vi "Application Memory Monitor.vi"() -> ()   [LabVIEW 2016]
uses:
  <vilib>/Utility/error.llb/DialogType.ctl
  SLL Queued State Machine/Queue Driver/Create Queue.vi
  SLL Queued State Machine/Queue Driver/Enqueue an Item to Queue.vi
  SLL Queued State Machine/Queue Driver/Dequeue Queue.vi
  SLL Queued State Machine/Queue Driver/Enqueue N Items.vi
  SLL Queued State Machine/Queue Driver/Flush Queue.vi
  SLL Queued State Machine/Queue Driver/Release Queue.vi
  SLL Queued State Machine/SLL QSM.lvlib
panel:
  in  "Start":bool
  in  "Sampling Rate (s)":dbl=1.0
  in  "Application Image Name":string="LabVIEW"
  out "Waveform Chart":T1(graph)
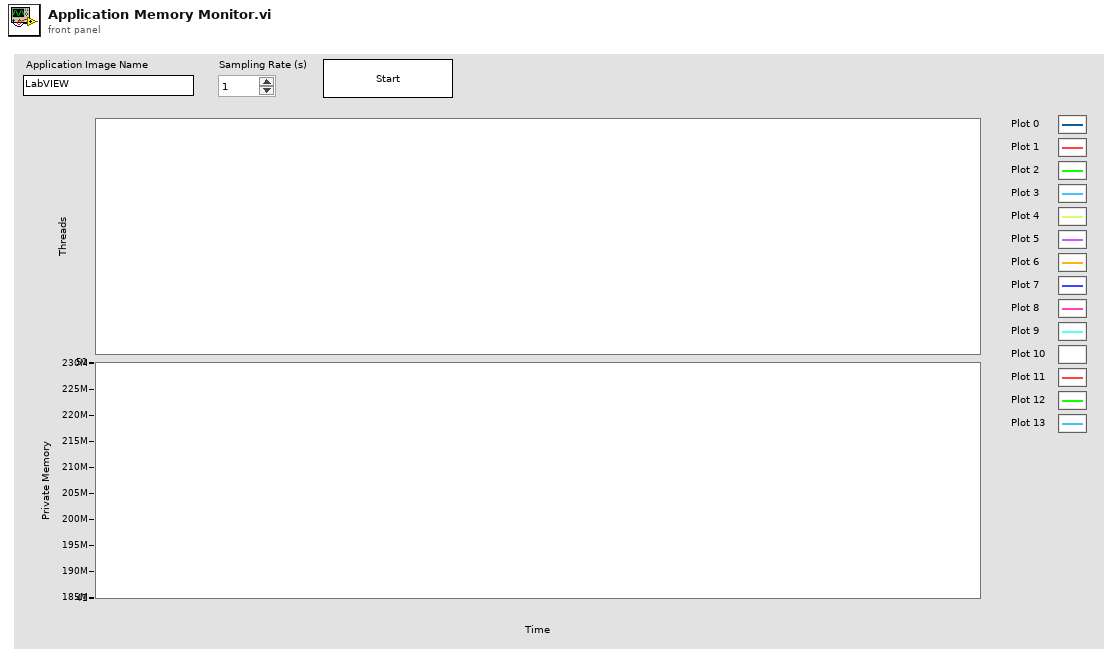
[diagram p1: front panel]
types:
  T1 = cluster{"Thread Count":i32, "PrivateMemorySize64":i64}
  T2 = cluster{"Flags":cluster{"Source Code?":bool, "Running?":bool}, "Application Name":string, "Ref":cluster{"ProcessMain":refnum<k24>, "UserProcess":refnum<k24>, "Threads":refnum<k24>}, "Sampling Rate (ms)":i32}
  T3 = cluster{"Thread Count":i32, "PrivateMemorySize64":i64}[]
  T4 = typedef "DialogType.ctl" = u16
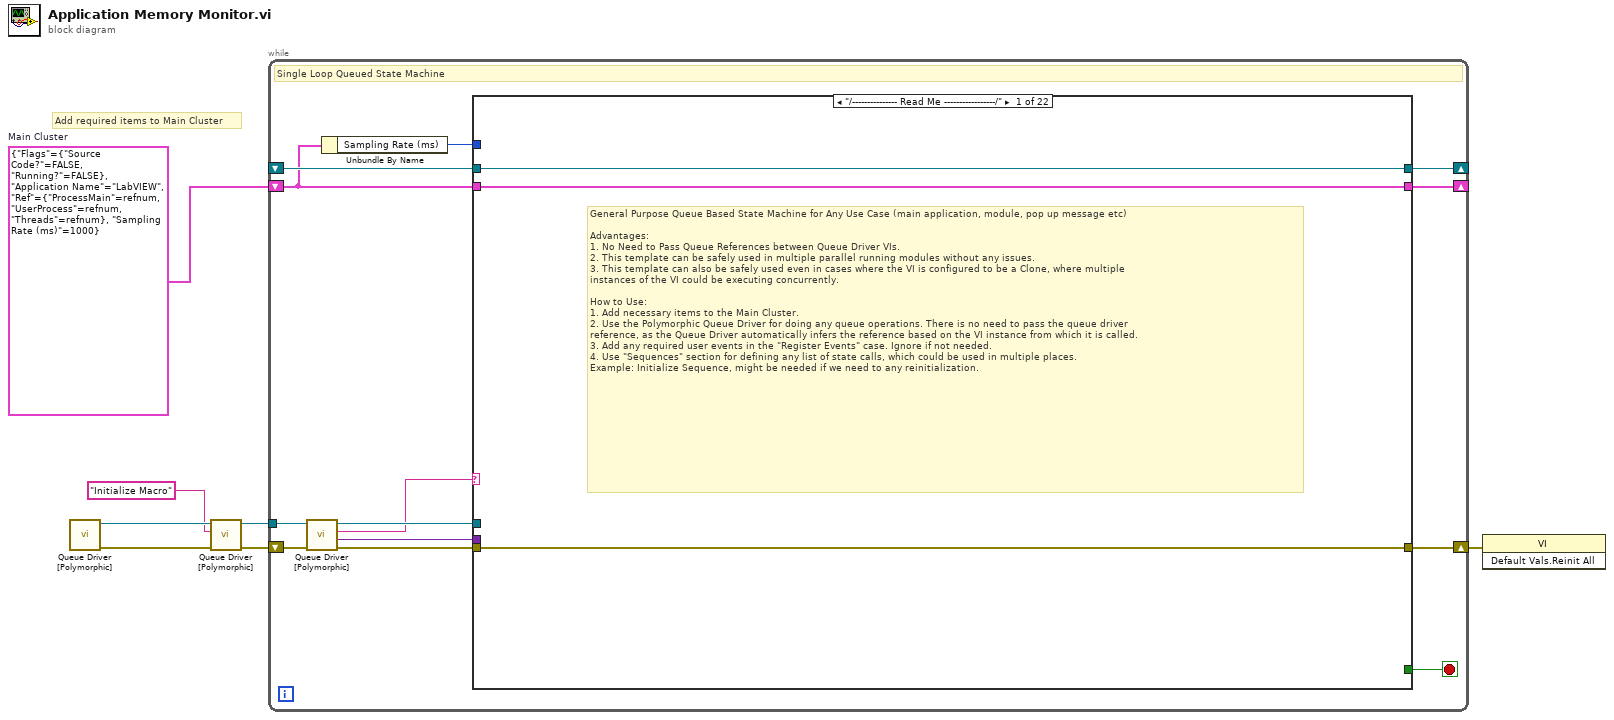
[diagram p0: block diagram]
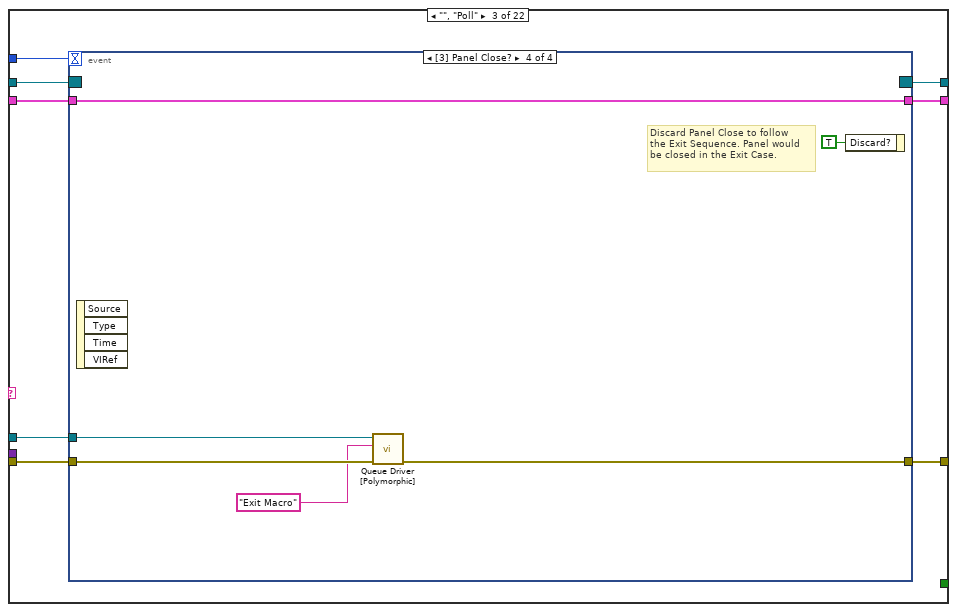
[diagram p3: hidden frame]
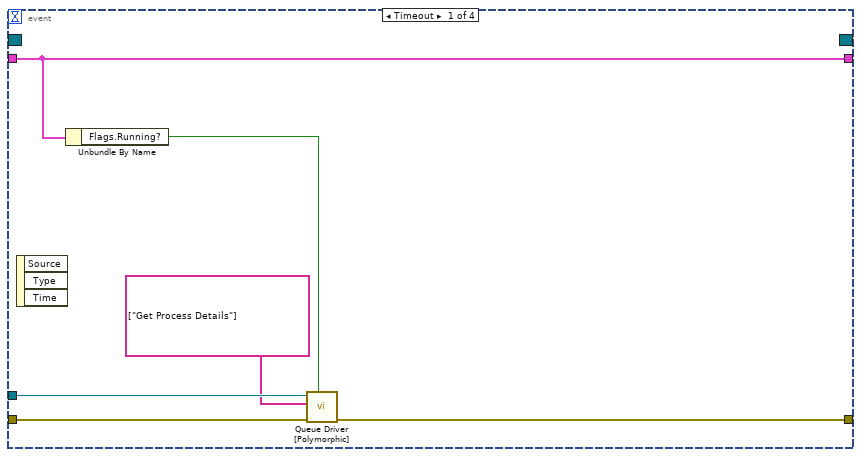
[diagram p4: hidden frame]
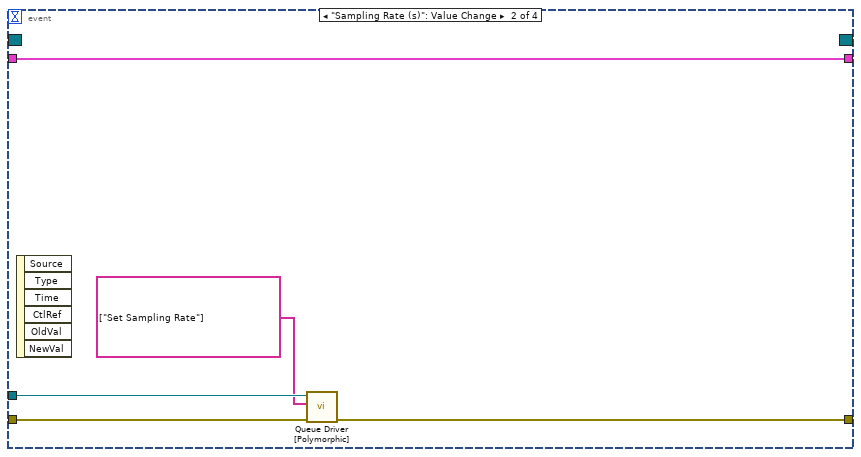
[diagram p5: hidden frame]
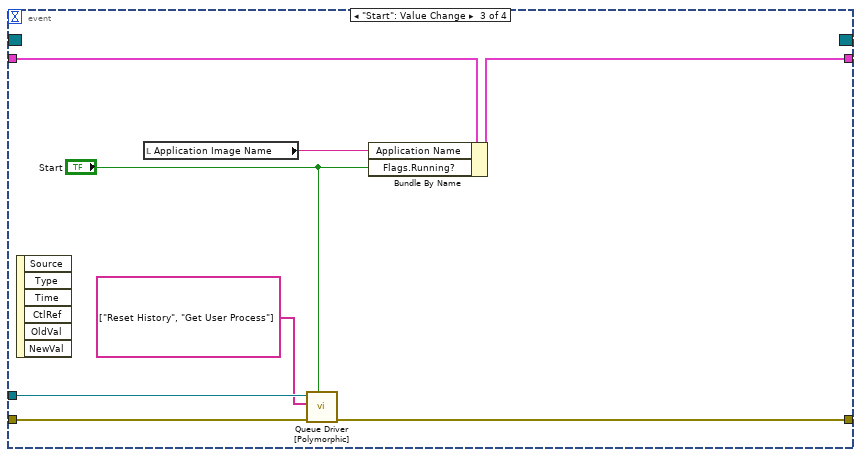
[diagram p6: hidden frame]
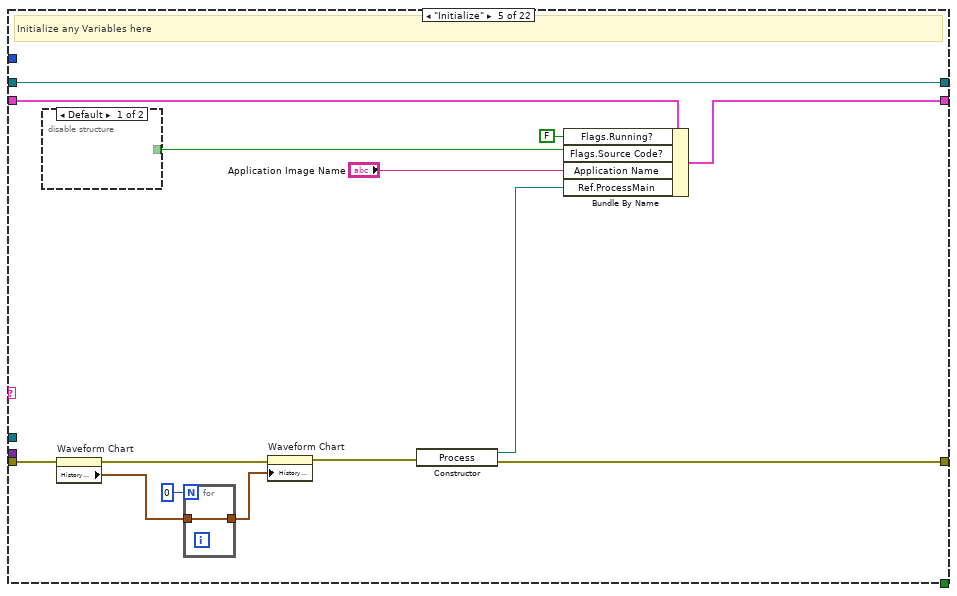
[diagram p8: hidden frame]
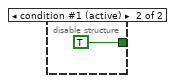
[diagram p9: hidden frame]
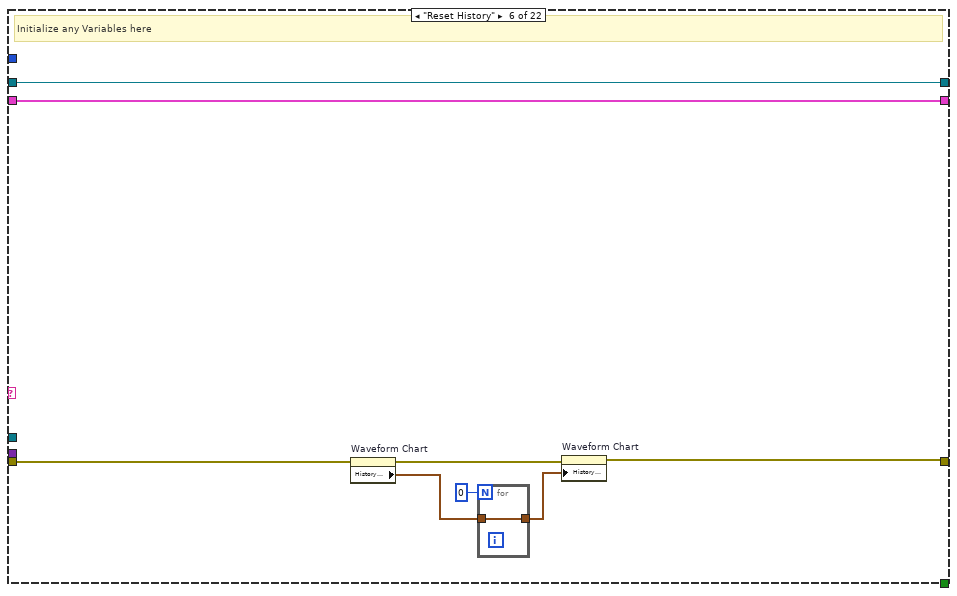
[diagram p10: hidden frame]
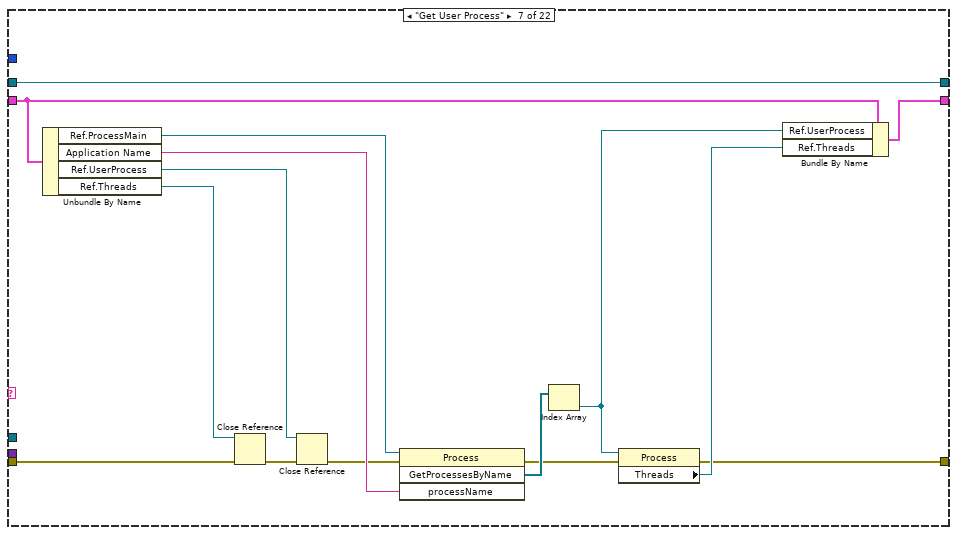
[diagram p11: hidden frame]
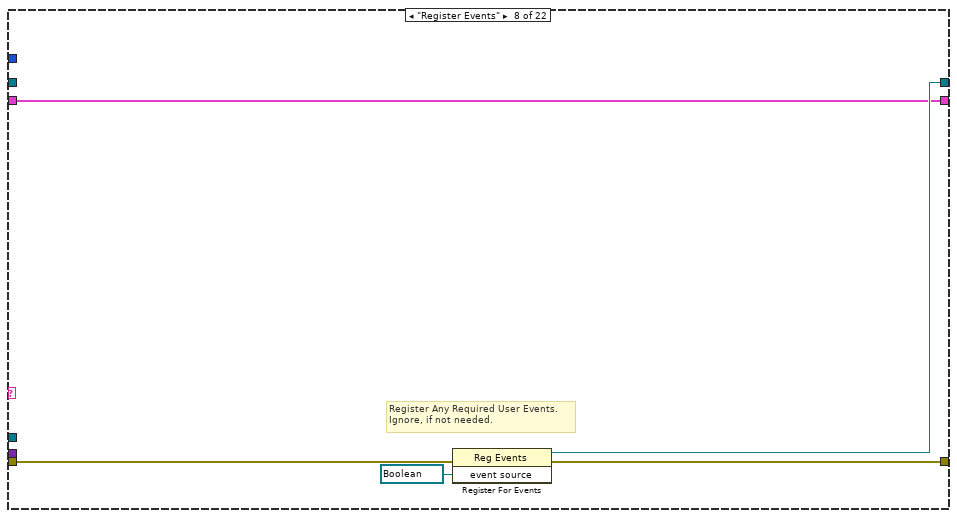
[diagram p12: hidden frame]
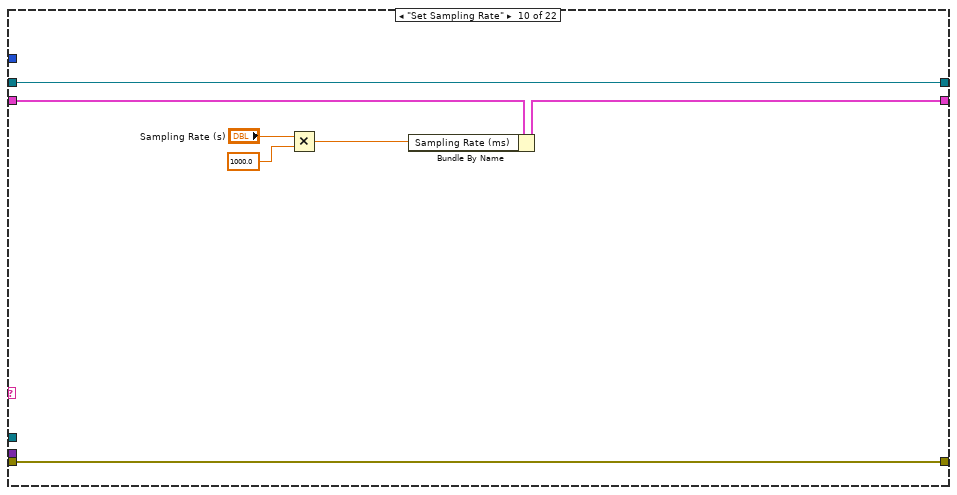
[diagram p14: hidden frame]
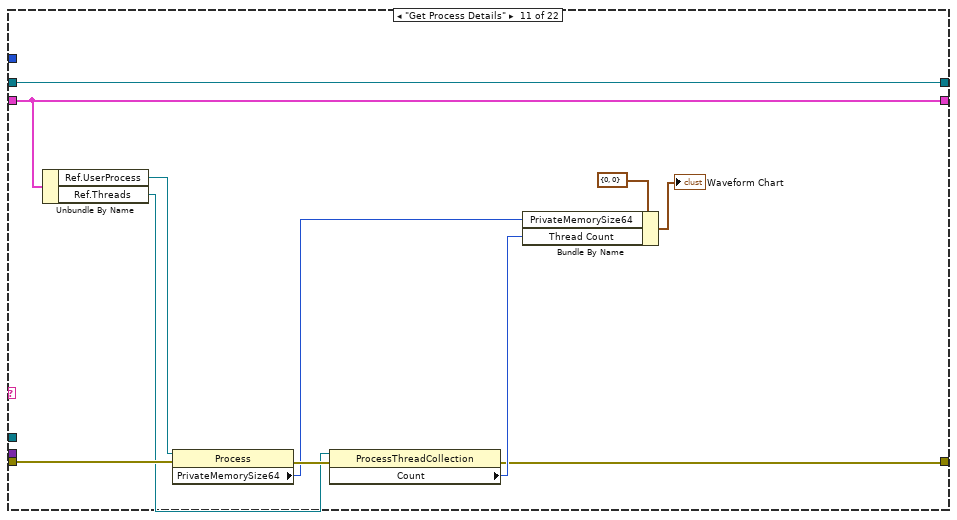
[diagram p15: hidden frame]
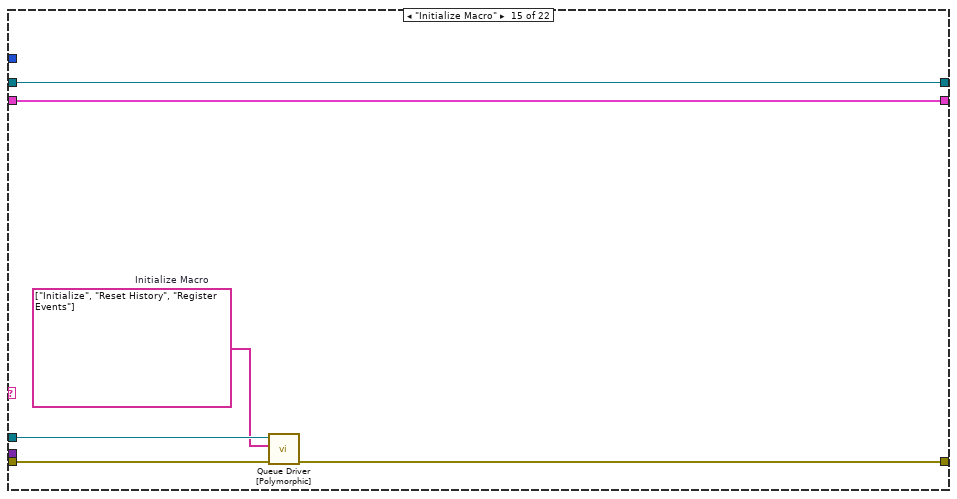
[diagram p19: hidden frame]
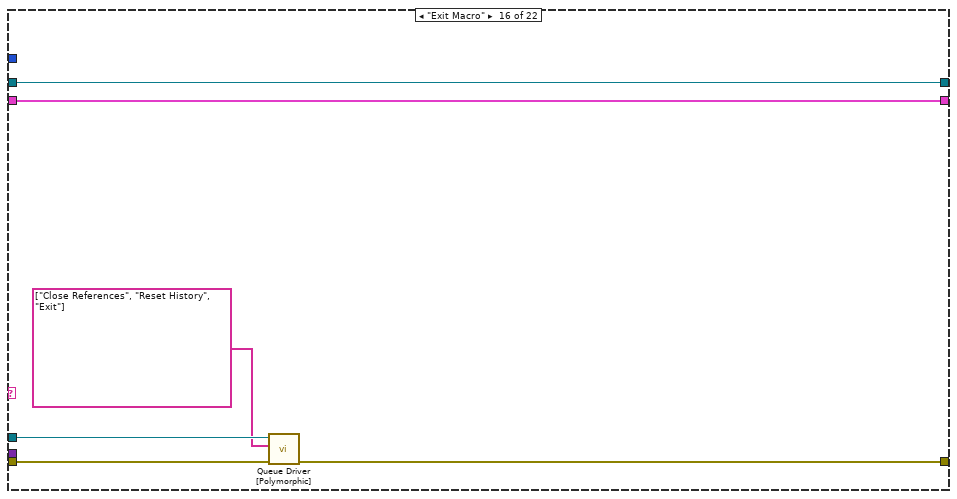
[diagram p20: hidden frame]
diagram:
  w7 = T2 {"Flags"={"Source Code?"=FALSE, "Running?"=FALSE}, "Application Name"="LabVIEW", "Ref"={"ProcessMain"=refnum, "UserProcess"=refnum, "Threads"=refnum}, "Sampling Rate (ms)"=1000}  # Main Cluster
  # "Add required items to Main Cluster"
  n1 = call-poly "Queue Driver [Polymorphic].vi"() -> ("Error Out"=w5:errorcluster, "Queue Ref"=w4:refnum<queue>)  [unwired: 10 in]
  n2 = call-poly "Queue Driver [Polymorphic].vi"("Error In"=w5, "Item to Add"="Initialize Macro", "Queue Ref In"=w4) -> ("Error Out"=w6:errorcluster, "Queue Ref Out"=w2:refnum<queue>)  [unwired: 7 in]
  n3 = while "SLL Queued State Machine" {
    shift-right: [w18] -> w1
    shift-left: w6 -> [w20]
    shift-right: [w15] -> _
    shift-left: _ -> [w14]
    shift-right: [w13] -> _
    shift-left: w7 -> [w11]
    tunnel: w2 -> [w9]
    stop <- w17 stop-if-true
    # "Single Loop Queued State Machine"
    n4 = call-poly "Queue Driver [Polymorphic].vi"("Error In"=w20, "Queue Ref In"=w9) -> ("Error Out"=w19:errorcluster, "Data"=w8:variant, "Dequeue"=w12:string, "Queue Ref Out"=w16:refnum<queue>)  [unwired: 6 in]
    n5 = Unbundle By Name(w11) -> ("Sampling Rate (ms)"=w10:i32)
    n6 = case "QSM Case Structure" shown="\"/--------------- Read Me -----------------/\"" w12 {
      selector: w12 -> [_ _ _ _ _ _ _ _ _ _ _ _ _ _ _ _ _ w153 _ _ _ _]
      tunnel: w19 -> [w23 w26 w33 w62 w69 w84 w99 w107 w110 w117 w126 w131 w134 w137 w141 w147 w152 w156 w168 w171 w175 w193]
      tunnel: [w23 w26 w34 w62 w71 w82 w93 w106 w110 w117 w118 w131 w134 w137 w140 w146 w152 w159 w166 w171 w174 w189] -> w18
      tunnel: [_ _ _ _ _ _ _ _ _ _ _ _ _ _ _ _ _ _ _ _ _ TRUE] -> w17
      tunnel: [w22 w25 w32 w61 w76 w86 w102 w105 w109 w116 w128 w130 w133 w136 w143 w149 w151 w162 w165 w170 w180 w192] -> w15
      tunnel: w14 -> [w22 w25 w31 w61 w76 w86 w102 _ w109 w116 w128 w130 w133 w136 w143 w149 w151 w162 w165 w170 w180 w192]
      tunnel: [w21 w24 w29 w60 w73 w85 w96 w104 w108 w112 w127 w129 w132 w135 w142 w148 w150 w161 w164 w169 w179 w191] -> w13
      tunnel: w11 -> [w21 w24 w30 w60 w74 w85 w97 w104 w108 w115 w127 w129 w132 w135 w142 w148 w150 w161 w164 w169 w179 w191]
      tunnel: w10 -> [_ _ w28 _ _ _ _ _ _ _ _ _ _ _ _ _ _ _ _ _ _ _]
      tunnel: w16 -> [_ _ w27 _ _ _ _ _ _ _ _ _ _ _ w139 w145 _ _ _ _ _ w182]
      tunnel: w8 -> [_ _ _ _ _ _ _ _ _ _ _ _ _ _ _ _ _ _ _ _ _ _]
      frame "/--------------- Read Me -----------------/" {
        # "General Purpose Queue Based State Machine for Any Use Case (main application, module, pop up message etc)\n\nAdvantages:\n1. No Need to Pass Queue References between Queue Driver VIs.\n2. This template can be safely used in multiple parallel running modules without any issues.\n3. This template can also be safely used even in cases where the VI is configured to be a Clone, where multiple \ninstances of the VI could be executing concurrently.\n\nHow to Use:\n1. Add necessary items to the Main Cluster.\n2. Use the Polymorphic Queue Driver for doing any queue operations. There is no need to pass the queue driver\nreference, as the Queue Driver automatically infers the reference based on the VI instance from which it is called.\n3. Add any required user events in the \"Register Events\" case. Ignore if not needed.\n4. Use \"Sequences\" section for defining any list of state calls, which could be used in multiple places. \nExample: Initialize Sequence, might be needed if we need to any reinitialization."
      }
      frame "/------------------ Poll -------------------/" {
      }
      frame "", "Poll" {
        n7 = event shown="[3] Panel Close?" {
          selector: w31 -> [_ _ _ _]
          dyn-events: [_ _ _ _] -> w32
          timeout: w28 -> [_ _ _ _]
          tunnel: [w39 w43 w51 w58] -> w34
          tunnel: w33 -> [w40 w44 w52 w59]
          tunnel: w30 -> [w36 w45 w53 w57]
          tunnel: [w36 w45 w48 w57] -> w29
          tunnel: w27 -> [w38 w42 w50 w54]
          event Timeout {
            n8 = event-data() -> ()  [unwired: 1 in, 3 out]
            n9 = Unbundle By Name(w36) -> ("Flags.Running?"=w35:bool)
            n10 = call-poly "Queue Driver [Polymorphic].vi"("Add to Queue? (T)"=w35, "Error In"=w40, "Enqueue N"=string[] ["Get Process Details"], "Queue Ref In"=w38) -> ("Error Out"=w39:errorcluster)  [unwired: 6 in, 1 out]
          }
          event "Sampling Rate (s)": Value Change {
            n11 = event-data() -> ()  [unwired: 1 in, 6 out]
            n12 = call-poly "Queue Driver [Polymorphic].vi"("Error In"=w44, "Enqueue N"=string[] ["Set Sampling Rate"], "Queue Ref In"=w42) -> ("Error Out"=w43:errorcluster)  [unwired: 7 in, 1 out]
          }
          event "Start": Value Change {
            n13 = event-data() -> ()  [unwired: 1 in, 6 out]
            n14 = local read "Application Image Name"() -> (w46:string)
            n15 = call-poly "Queue Driver [Polymorphic].vi"("Add to Queue? (T)"="Start", "Error In"=w52, "Enqueue N"=string[] ["Reset History", "Get User Process"], "Queue Ref In"=w50) -> ("Error Out"=w51:errorcluster)  [unwired: 6 in, 1 out]
            n16 = Bundle By Name(cluster=w53, "Application Name"=w46, "Flags.Running?"="Start") -> (w48:T2)
          }
          event Panel Close? {
            # "Discard Panel Close to follow\nthe Exit Sequence. Panel would\nbe closed in the Exit Case."
            n17 = event-data() -> ()  [unwired: 1 in, 4 out]
            n18 = call-poly "Queue Driver [Polymorphic].vi"("Error In"=w59, "Item to Add"="Exit Macro" ("Enqueue"), "Queue Ref In"=w54) -> ("Error Out"=w58:errorcluster)  [unwired: 7 in, 1 out]
            n19 = event-data("Discard?"=TRUE) -> ()  [unwired: 1 in, 1 out]
          }
        }
      }
      frame "/--------------- Initialize -----------------/" {
      }
      frame "Initialize" {
        # "Initialize any Variables here"
        n20 = disable-structure shown="Default" {
          disable-tunnel: [_ TRUE] -> w75
          frame condition #0 {
          }
          frame condition #1 (active) {
          }
        }
        n21 = property on="Waveform Chart" class="WFChart (strict)"(error in=w69) -> (error out=w68:errorcluster, "History Data"=w65:T3)  [unwired: 1 in, 1 out]
        n22 = for {
          N: 0 -> [_]
          tunnel: w65 -> [w77]
          tunnel: [w77] -> w64
        }
        n23 = property on="Waveform Chart" class="WFChart (strict)"(error in=w68, "History Data"=w64) -> (error out=w67:errorcluster)  [unwired: 1 in, 1 out]
        n24 = constructor class="Process"(error in=w67) -> (reference out=w70:refnum<k24>, error out=w71:errorcluster)  [unwired: 2 in, 1 out]
        n25 = Bundle By Name(cluster=w74, "Flags.Running?"=FALSE, "Flags.Source Code?"=w75, "Application Name"="Application Image Name", "Ref.ProcessMain"=w70) -> (w73:T2)
      }
      frame "Reset History" {
        # "Initialize any Variables here"
        n26 = property on="Waveform Chart" class="WFChart (strict)"(error in=w84) -> (error out=w83:errorcluster, "History Data"=w80:T3)  [unwired: 1 in, 1 out]
        n27 = for {
          N: 0 -> [_]
          tunnel: w80 -> [w87]
          tunnel: [w87] -> w79
        }
        n28 = property on="Waveform Chart" class="WFChart (strict)"(error in=w83, "History Data"=w79) -> (error out=w82:errorcluster)  [unwired: 1 in, 1 out]
      }
      frame "Get User Process" {
        n29 = Unbundle By Name(w97) -> ("Ref.ProcessMain"=w100:refnum<k24>, "Application Name"=w98:string, "Ref.UserProcess"=w89:refnum<k24>, "Ref.Threads"=w88:refnum<k24>)
        n30 = Close Reference(reference=w88, error in (no error)=w99) -> (error out=w91:errorcluster)
        n31 = Close Reference(reference=w89, error in (no error)=w91) -> (error out=w90:errorcluster)
        n32 = invoke class="Process" method="GetProcessesByName"(reference=w100, error in=w90, "processName"=w98) -> (error out=w92:errorcluster, "GetProcessesByName"=w101:refnum<k24>[])  [unwired: 1 in, 2 out]
        n33 = Index Array(array=w101) -> (element=w95:refnum<k24>)  [unwired: 1 in]
        n34 = property class="Process"(reference=w95, error in=w92) -> (error out=w93:errorcluster, "Threads"=w94:refnum<k24>)  [unwired: 1 out]
        n35 = Bundle By Name(cluster=w97, "Ref.UserProcess"=w95, "Ref.Threads"=w94) -> (w96:T2)
      }
      frame "Register Events" {
        # "Register Any Required User Events. \nIgnore, if not needed."
        n36 = register-events(error in=w107, refnum<vi> refnum ("event source")) -> (reference out=w105:refnum<event-registration>, error out=w106:errorcluster)  [unwired: 1 in]
      }
      frame "/---------- Process Monitor ----------/" {
      }
      frame "Set Sampling Rate" {
        n37 = Multiply(x="Sampling Rate (s)", y=1000.0) -> (x*y=w111:dbl)
        n38 = Bundle By Name(cluster=w115, "Sampling Rate (ms)"=w111) -> (w112:T2)
      }
      frame "Get Process Details" {
        n39 = Unbundle By Name(w127) -> ("Ref.UserProcess"=w125:refnum<k24>, "Ref.Threads"=w122:refnum<k24>)
        n40 = property class="Process"(reference=w125, error in=w126) -> (error out=w124:errorcluster, "PrivateMemorySize64"=w121:i64)  [unwired: 1 out]
        n41 = property class="ProcessThreadCollection"(reference=w122, error in=w124) -> (error out=w118:errorcluster, "Count"=w120:i32)  [unwired: 1 out]
        n42 = Bundle By Name(cluster=T1 {"Thread Count"=0, "PrivateMemorySize64"=0}, "PrivateMemorySize64"=w121, "Thread Count"=w120) -> (→"Waveform Chart":T1)
      }
      frame "/-------------- User Interface --------------/" {
        # "Duplicate this case to create additional case splitters for readability"
      }
      frame "Update UI" {
        # "Update Front Panel Controls in this Case"
      }
      frame "/----------------- Macros -----------------/" {
      }
      frame "Initialize Macro" {
        w138 = string[] ["Initialize", "Reset History", "Register Events"]  # Initialize Macro
        n43 = call-poly "Queue Driver [Polymorphic].vi"("Error In"=w141, "Enqueue N"=w138, "Queue Ref In"=w139) -> ("Error Out"=w140:errorcluster)  [unwired: 7 in, 1 out]
      }
      frame "Exit Macro" {
        n44 = call-poly "Queue Driver [Polymorphic].vi"("Error In"=w147, "Enqueue N"=string[] ["Close References", "Reset History", "Exit"], "Queue Ref In"=w145) -> ("Error Out"=w146:errorcluster)  [unwired: 7 in, 1 out]
      }
      frame "/-------------- Error Handler--------------/" {
      }
      frame Default {
        # "Undefined Case/Spelling Errors - Show Message to Developer"
        n45 = property class="VI"(error in=w156) -> (error out=w155:errorcluster, "Name"=w154:string)  [unwired: 1 in, 1 out]
        n46 = Format Into String(format string="\"%s\" in the VI - %s" ("message"), initial string="Undefined case - ", error in=w155, w153, w154) -> (resulting string=w157:string, error out=w159:errorcluster)
        n47 = One Button Dialog(message=w157) -> ()  [unwired: 1 in, 1 out]
      }
      frame "Error" {
        w163 = T4 2 items=["no dialog", "OK message", "continue or stop message", "OK message + warnings", "continue/stop + warnings"] ("type of dialog (OK msg:1)")
        # "Handle the Error"
        n48 = call <vilib>:"Simple Error Handler.vi"("type of dialog (OK msg:1)"=w163, "error in (no error)"=w168) -> ("error out"=w167:errorcluster)  [unwired: 3 in, 4 out]
        n49 = call <vilib>:"Clear Errors.vi"("error in (no error)"=w167) -> ("error out"=w166:errorcluster)  [unwired: 5 in, 1 out]
      }
      frame "/------------------- Exit --------------------/" {
      }
      frame "Close References" {
        n50 = Unbundle By Name(w179) -> ("Ref.ProcessMain"=w176:refnum<k24>, "Ref.UserProcess"=w177:refnum<k24>, "Ref.Threads"=w172:refnum<k24>)
        n51 = Close Reference(reference=w172, error in (no error)=w175) -> (error out=w173:errorcluster)
        n52 = Close Reference(reference=w177, error in (no error)=w173) -> (error out=w178:errorcluster)
        n53 = Close Reference(reference=w176, error in (no error)=w178) -> (error out=w174:errorcluster)
      }
      frame "Exit" {
        n54 = call-poly "Queue Driver [Polymorphic].vi"("Error In"=w193, "Queue Ref In"=w182) -> ("Error Out"=w194:errorcluster, "Queue Ref Out"=w181:refnum<queue>)  [unwired: 7 in, 1 out]
        n55 = Unbundle By Name(w191) -> ("Flags.Source Code?"=w184:bool)
        n56 = call-poly "Queue Driver [Polymorphic].vi"("Error In"=w194, "Queue Ref In"=w181) -> ("Error Out"=w190:errorcluster)  [unwired: 9 in]
        n57 = Call Chain() -> (call chain=w188:string[])
        n58 = Array Size(array=w188) -> (size(s)=w187:i32)
        n59 = Equal?(x=w187, y=1) -> (x = y?=w185:bool)
        n60 = And(x=w184, y=w185) -> (x .and. y?=w183:bool)
        n61 = case "Skip Panel Close when in Source\nCode and is the top most caller" shown="False" w183 {
          tunnel: w190 -> [w197 w199]
          tunnel: [w198 w199] -> w189
          frame False {
            # "Close Panel"
            n62 = invoke class="VI" method="FP.Close"() -> (error out=w196:errorcluster)  [unwired: 3 in, 2 out]
            n63 = Merge Errors(w197, w196) -> (w198:errorcluster)
          }
          frame True {
            # "Do Not Close Panel"
          }
        }
      }
    }
  }
  n64 = invoke class="VI" method="Default Vals.Reinit All"(error in=w1) -> ()  [unwired: 2 in, 3 out]
